vi "MotorDirectionHandler (SubVI).vi"(8 "Speed Setpoint":dbl, 10 "Movement":T1(ring), 11 "Motor Number":T2(ring)) -> (3 "Speed Setpoint Output":dbl)   [LabVIEW 2017]
panel:
  # "VI Name: MotorDirectionHandler (SubVI).vi\nAuthor: Steven Lee\n\nPurpose: \nThis VI provides the speed setpoint required for PID controller's input, given that the following data is provided:\n\n* Motor Number\n* Movement Direction\n* Current speed setpoint"
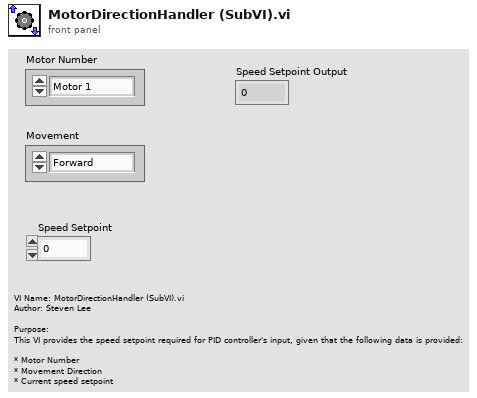
[diagram p1: front panel]
types:
  T1 = enum16{"Forward", "Backward", "Left", "Right", "Rotate Left", "Rotate Right"}
  T2 = enum16{"Motor 1", "Motor 2", "Motor 3", "Motor 4"}
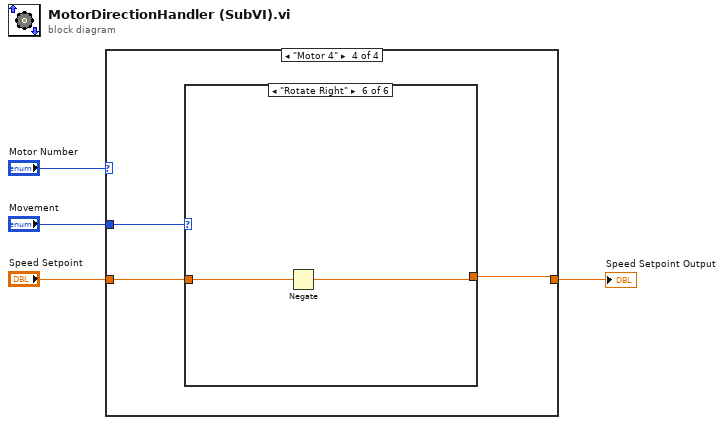
[diagram p0: block diagram]
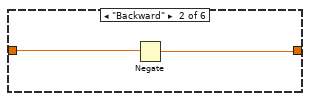
[diagram p4: hidden frame]
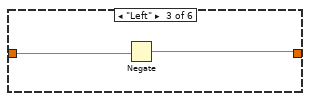
[diagram p5: hidden frame]
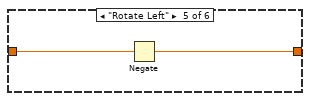
[diagram p7: hidden frame]
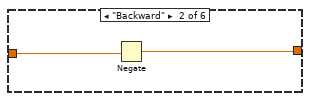
[diagram p9: hidden frame]
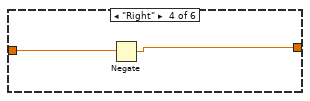
[diagram p11: hidden frame]
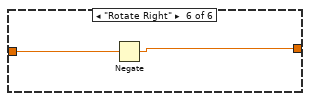
[diagram p13: hidden frame]
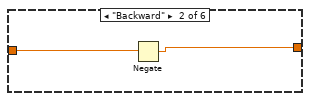
[diagram p15: hidden frame]
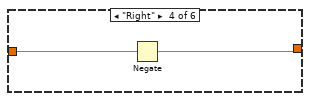
[diagram p17: hidden frame]
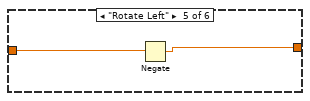
[diagram p18: hidden frame]
diagram:
  n1 = case shown="\"Motor 4\"" "Motor Number" {
    tunnel: "Speed Setpoint" -> [w7 w18 w30 w42]
    tunnel: [w6 w17 w29 w41] -> w3
    tunnel: "Movement" -> [w5 w19 w31 w43]
    frame "Motor 1", Default {
      n2 = case shown="\"Rotate Right\"" w5 {
        tunnel: w7 -> [w8 w10 w12 w13 w15 w16]
        tunnel: [w8 w9 w11 w13 w14 w16] -> w6
        frame "Forward", Default {
        }
        frame "Backward" {
          n3 = Negate(x=w10) -> (-x=w9:dbl)
        }
        frame "Left" {
          n4 = Negate(x=w12) -> (-x=w11:dbl)
        }
        frame "Right" {
        }
        frame "Rotate Left" {
          n5 = Negate(x=w15) -> (-x=w14:dbl)
        }
        frame "Rotate Right" {
        }
      }
    }
    frame "Motor 2" {
      n6 = case shown="\"Forward\", Default" w19 {
        tunnel: [w20 w21 w23 w24 w26 w27] -> w17
        tunnel: w18 -> [w20 w22 w23 w25 w26 w28]
        frame "Forward", Default {
        }
        frame "Backward" {
          n7 = Negate(x=w22) -> (-x=w21:dbl)
        }
        frame "Left" {
        }
        frame "Right" {
          n8 = Negate(x=w25) -> (-x=w24:dbl)
        }
        frame "Rotate Left" {
        }
        frame "Rotate Right" {
          n9 = Negate(x=w28) -> (-x=w27:dbl)
        }
      }
    }
    frame "Motor 3" {
      n10 = case shown="\"Forward\", Default" w31 {
        tunnel: [w32 w33 w35 w36 w38 w40] -> w29
        tunnel: w30 -> [w32 w34 w35 w37 w39 w40]
        frame "Forward", Default {
        }
        frame "Backward" {
          n11 = Negate(x=w34) -> (-x=w33:dbl)
        }
        frame "Left" {
        }
        frame "Right" {
          n12 = Negate(x=w37) -> (-x=w36:dbl)
        }
        frame "Rotate Left" {
          n13 = Negate(x=w39) -> (-x=w38:dbl)
        }
        frame "Rotate Right" {
        }
      }
    }
    frame "Motor 4" {
      n14 = case shown="\"Rotate Right\"" w43 {
        tunnel: [w44 w45 w47 w49 w50 w51] -> w41
        tunnel: w42 -> [w44 w46 w48 w49 w50 w52]
        frame "Forward", Default {
        }
        frame "Backward" {
          n15 = Negate(x=w46) -> (-x=w45:dbl)
        }
        frame "Left" {
          n16 = Negate(x=w48) -> (-x=w47:dbl)
        }
        frame "Right" {
        }
        frame "Rotate Left" {
        }
        frame "Rotate Right" {
          n17 = Negate(x=w52) -> (-x=w51:dbl)
        }
      }
    }
  }
  "Speed Setpoint Output" <- w3
